vi "trim data.vi"(1 "rect":T1, 2 "source graph":cluster{"x":dbl[], "y":dbl[]}) -> (0 "graph":cluster{dbl[], dbl[]})   [LabVIEW 2009]
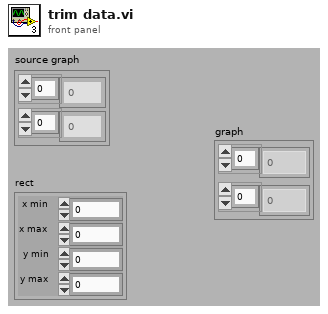
[diagram p1: front panel]
types:
  T1 = cluster{"x min":dbl, "x max":dbl, "y min":dbl, "y max":dbl}
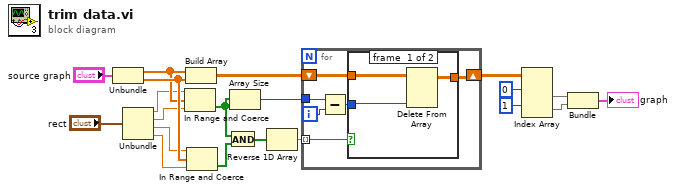
[diagram p0: block diagram]
diagram:
  n1 = Unbundle("source graph") -> ("x"=w3:dbl[], "y"=w8:dbl[])
  n2 = Unbundle("rect") -> ("x min"=w1:dbl, "x max"=w2:dbl, "y min"=w4:dbl, "y max"=w5:dbl)
  n3 = In Range and Coerce(upper limit=w1, x=w3, lower limit=w2) -> (In Range?=w16:bool[])  [unwired: 1 out]
  n4 = Build Array(w3, w8) -> (w17:dbl[][])
  n5 = In Range and Coerce(upper limit=w4, x=w8, lower limit=w5) -> (In Range?=w20:bool[])  [unwired: 1 out]
  n6 = And(x=w16, y=w20) -> (x .and. y?=w19:bool[])
  n7 = Array Size(array=w16) -> (size(s)=w15:i32)
  n8 = Reverse 1D Array(array=w19) -> (reversed array=w18:bool[])
  n9 = for {
    tunnel: w18 -> [w24] mode=indexing
    shift-right: [w22] -> w14
    shift-left: w17 -> [w23]
    tunnel: w15 -> [w26]
    i -> [w25]
    n10 = Subtract(x=w26, y=w25) -> (x-y=w21:i32)
    n11 = case shown="False" w24 {
      tunnel: w23 -> [w29 w30]
      tunnel: [w27 w30] -> w22
      tunnel: w21 -> [w28 _]
      frame #0 {
        n12 = Delete From Array(array=w29, index (col)=w28) -> (array with subset deleted=w27:dbl[][])  [unwired: 2 in, 1 out]
      }
      frame #1 {
      }
    }
  }
  n13 = Index Array(array=w14, index (row) #1=0 ("disabled index (col)"), index (row) #2=1 ("index (row)")) -> (element #1=w11:dbl[], element #2=w10:dbl[])  [unwired: 2 in]
  n14 = Bundle(w11, w10) -> (→"graph":cluster{dbl[], dbl[]})  [unwired: 1 in]
